vi "goal_loop.vi"(8 "error in":errorcluster, 11 "Micron config":T1) -> (0 "error out":errorcluster)   [LabVIEW 2014]
uses:
  initialization/micron_config.ctl
  manipulator/squiggle/Host/i2c_interface.ctl
  manipulator/squiggle/Host/fpga_reference.ctl
  testing/Micron params.ctl
  testing/stimulus.ctl
  testing/injection_point.ctl
  goal_loop_parms.ctl
  testing/mode_conrols.ctl
  testing/manipulator_cal.ctl
  asap/labview/testing/probe_calibration.ctl
  host/network_params.ctl
  cancellation/sq_control_params.ctl
  cancellation/decoupled_gain.ctl
  cancellation/estimation_controls.ctl
  <vilib>/Platform/TimedLoop/XDataNode/timing_clust.ctl
  <vilib>/Platform/TimedLoop/XDataNode/nitl_modes.ctl
  <vilib>/Platform/TimedLoop/XDataNode/wakeup.ctl
  testing/stimulate.vi
  <vilib>/Analysis/baseanly.llb/A x B.vi
  <vilib>/Analysis/baseanly.llb/A x Vector.vi
  initialization/micron_globals.vi
  <vilib>/Platform/TimedLoop/XDataNode/XDataNode.xnode
  <vilib>/Platform/TimedLoop/XDataNode/XDNodeRunTimeDep.lvlib
panel:
  in  "Sampling frequency":sgl=1000.0
  # "Locals:"
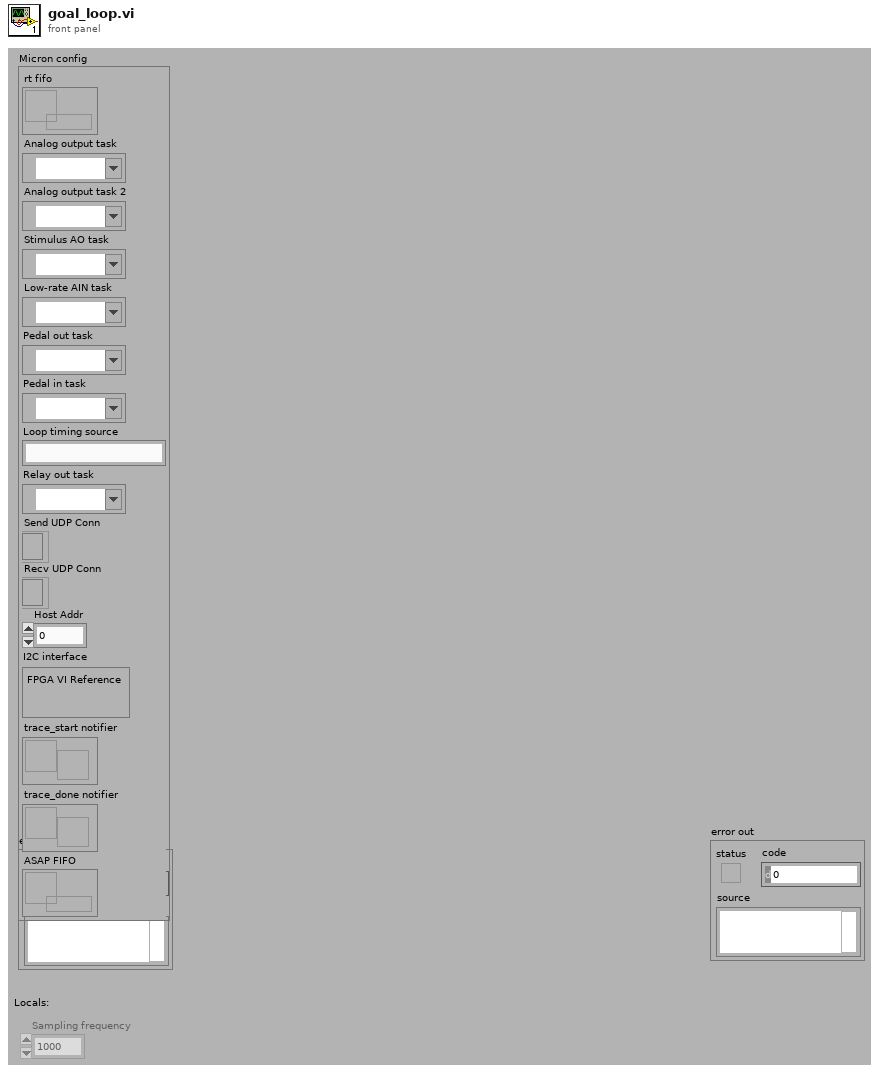
[diagram p1: front panel]
types:
  T1 = typedef "micron_config.ctl" = cluster{"rt fifo":refnum<k33>, "Analog output task":refnum<k21>, "Analog output task 2":refnum<k21>, "Stimulus AO task":refnum<k21>, "Low-rate AIN task":refnum<k21>, "Pedal out task":refnum<k21>, "Pedal in task":refnum<k21>, "Loop timing source":string, "Relay out task":refnum<k21>, "Send UDP Conn":refnum<k16>, "Recv UDP Conn":refnum<k16>, "Host Addr":u32, "I2C interface":T2, "trace_start notifier":refnum<notifier>, "trace_done notifier":refnum<notifier>, "ASAP FIFO":refnum<k33>}
  T2 = typedef "i2c_interface.ctl" = cluster{"FPGA VI Reference":T3}
  T3 = typedef "fpga_reference.ctl" = refnum<k20>
  T4 = typedef "Micron params.ctl" = cluster{"Stimulus":T5, "Goal Filter A":T7, "Mode controls":T8, "Manipulator type":enum16{"Current piezo", "Voltage piezo"}, "Manipulator calibration":T9, "Network":T11, "Goal Filter B":T7, "Cancellation":T12, "Transition time":sgl, "Estimation":T14}
  T5 = typedef "stimulus.ctl" = cluster{"Type":enum16{"Off", "Step", "Sine", "Triangle", "Arbitrary"}, "Phase":dbl, "Amplitude":sgl[], "Injection point":T6, "Closed loop":bool, "Offset":sgl[], "Tip -> world":bool, "Frequency":dbl, "Length":dbl}
  T6 = typedef "injection_point.ctl" = enum16{"Total pose", "V limiter", "Goal ", "Link position", "KF link position", "Inverse kin", "Link goal", "Link error", "Controller", "Output", "Drive", "Light"}
  T7 = typedef "goal_loop_parms.ctl" = cluster{"Speedup max":sgl, "Speedup thresh":sgl, "Speedup nonlin":sgl, "Filters":cluster{"Lower Fc":sgl, "Lower Q":sgl, "Scale factor":sgl, "Upper Fc":sgl, "Upper Q":sgl, "V limit":sgl, "V limit range":sgl}[]}
  T8 = typedef "mode_conrols.ctl" = cluster{"Hold":bool, "Cancellation":bool, "Goal filter":bool, "Trigger":bool}
  T9 = typedef "manipulator_cal.ctl" = cluster{"Tool offsets":sgl[][], "Tip light calibration":T10, "Handle light calibration":T10, "Base pivots":sgl[][], "Output pivots":sgl[][], "Length center":sgl, "Workspace height":sgl[], "Workspace diameter":sgl[], "Linearization":sgl[][], "Stack travel":sgl, "Saturation pos":sgl, "Inverse filters":cluster{"filter structure":enum32{"IIR 2nd Order", "IIR 4th Order"}, "Reverse Coefficients":dbl[], "Forward Coefficients":dbl[]}[]}
  T10 = typedef "probe_calibration.ctl" = sgl[][]
  T11 = typedef "network_params.ctl" = cluster{"Remote Host":string, "Send Status":bool, "Send Port":u16, "Recv Commands":bool, "Recv Port":u16}
  T12 = typedef "sq_control_params.ctl" = cluster{"KP":T13, "KI":sgl, "KD":T13, "Max vel":sgl, "Max acc":sgl, "Int error limit":sgl, "RCM gain":sgl, "Bypass":bool, "Degraded gain":sgl}
  T13 = typedef "decoupled_gain.ctl" = cluster{"XY":sgl, "Rxy":sgl, "Z":sgl, "Rz":sgl}
  T14 = typedef "estimation_controls.ctl" = cluster{"Link":cluster{"Measure noise":dbl[], "Process noise":dbl[], "Alt process noise":dbl[], "Alt turnoff cycles":i32, "Innovation limit":dbl[], "Residue threshold":dbl, "Enable":bool}, "Handle":cluster{"Measure noise":dbl[], "Process noise":dbl[], "State limits":dbl[], "Innovation limit":dbl[], "Prediction Lookahead":sgl, "Enable":bool}}
  T15 = typedef "XDNodeRunTimeDep.lvlib/timing_clust.ctl" = cluster{"Expected End [f-1]":u64, "Actual End [f-1]":u64, "Finished Late? [f-1]":bool, "Expected End [i-1]":u64, "Actual End [i-1]":u64, "Finished Late? [i-1]":bool, "Expected Start [i]":u64, "Actual Start [i]":u64, "Expected Start [f]":u64, "Actual Start [f]":u64, "Source Name":string, "Structure Name":string, "Period":i64, "Deadline":i64, "Offset":i64, "Start":i64, "Priority":i32, "Timeout":i32, "Mode":T16, "Wakeup Reason":T17, "Error":errorcluster, "Source Type":string, "Secondary Source Type":string, "Global End Time":u64, "Global Start Time":u64, "Frame Duration":u64, "Iteration Duration":u64, "Assigned CPU":i32, "I/O Scan Engine Mode":u32}
  T16 = typedef "XDNodeRunTimeDep.lvlib/nitl_modes.ctl" = enum32{"No Change", "Process missed periods, maintain original phase", "Discard missed periods, maintain original phase", "Process missed periods, ignore original phase", "Discard missed periods, ignore original phase"}
  T17 = typedef "XDNodeRunTimeDep.lvlib/wakeup.ctl" = enum32{"Normal", "Aborted", "Asynchronous wakeup", "Timing source error", "Timed loop error", "Timeout"}
  T18 = cluster{"Lower Fc":sgl, "Lower Q":sgl, "Scale factor":sgl, "Upper Fc":sgl, "Upper Q":sgl, "V limit":sgl, "V limit range":sgl}[]
  T19 = typedef "NI_Matrix.lvlib/RealMatrix.ctl" = dbl[][]
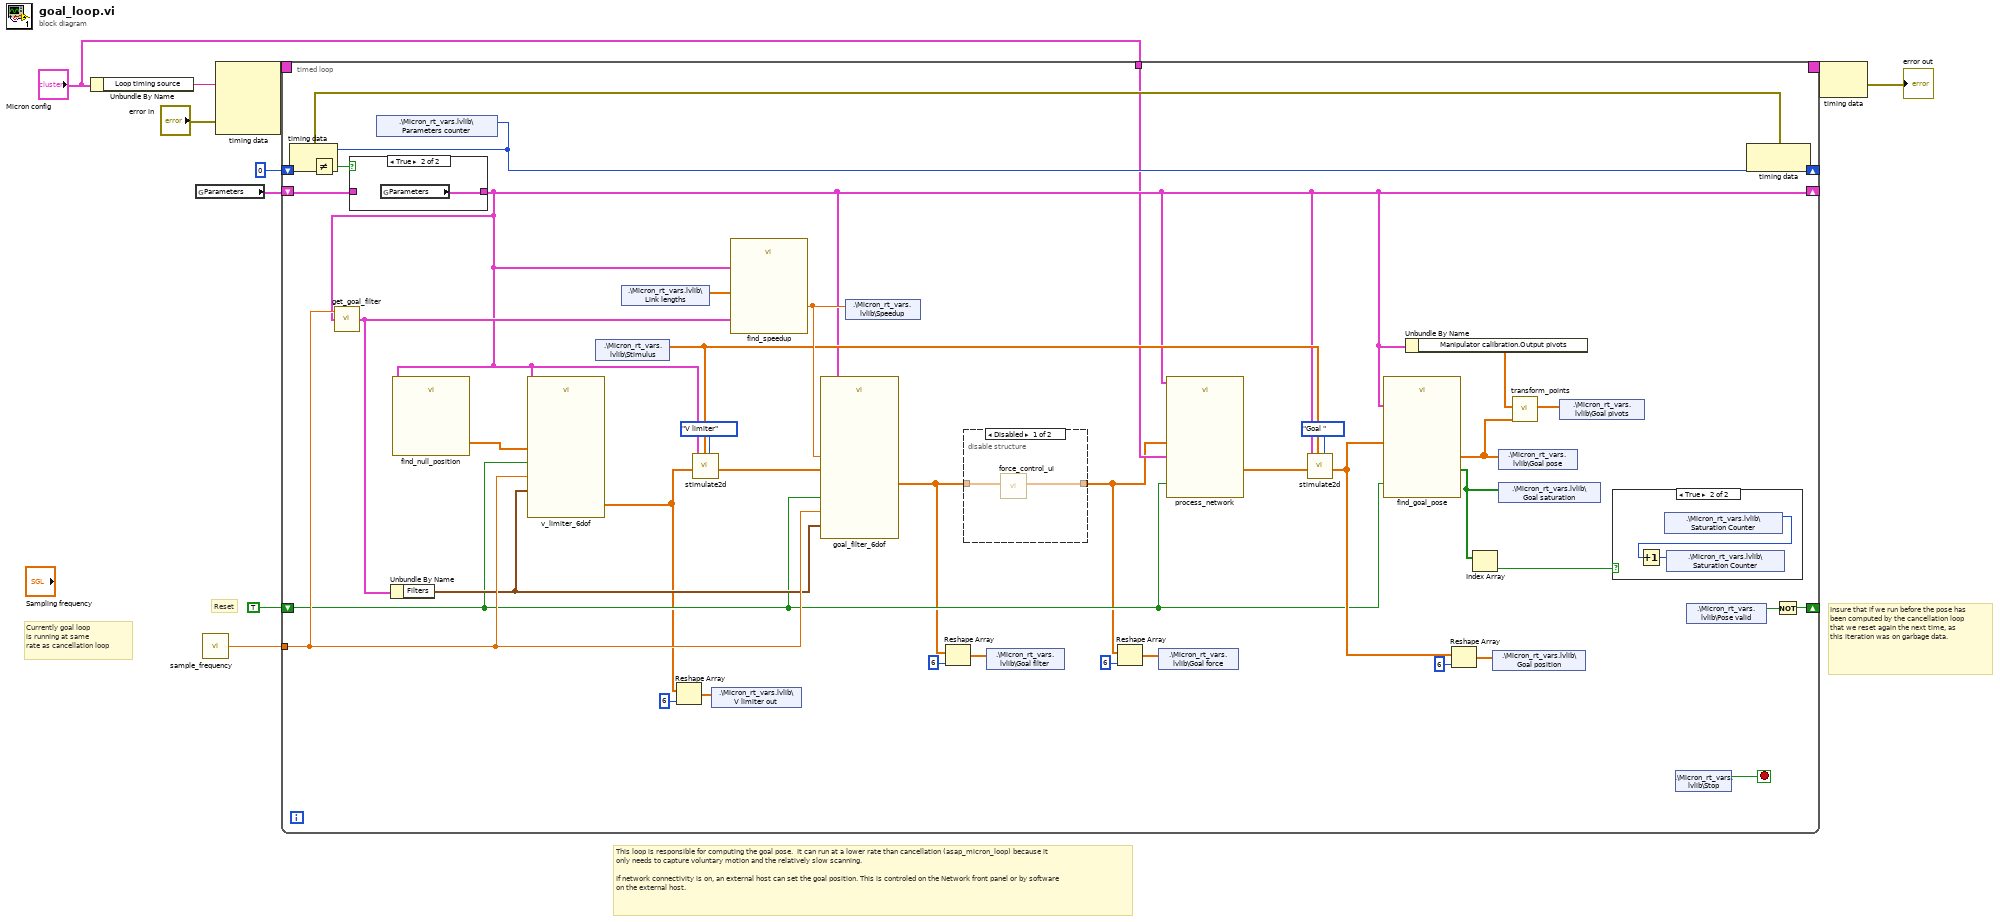
[diagram p0: block diagram]
diagram:
  # "Currently goal loop\nis running at same\nrate as cancellation loop"
  # "Reset"
  # "Insure that if we run before the pose has been computed by the cancellation loop that we reset again the next time, as this iteration was on garbage data."
  # "This loop is responsible for computing the goal pose.  It can run at a lower rate than cancellation (asap_micron_loop) because it only needs to capture voluntary motion and the relatively slow scanning.\n\nIf network connectivity is on, an external host can set the goal position. This is controled on the Network front panel or by software on the external host."
  n1 = Unbundle By Name("Micron config") -> ("Loop timing source"=w2:string)
  n2 = global read "micron_globals.vi" "Parameters"() -> (w4:T4)
  n3 = call "sample_frequency.vi"() -> ("Sample frequency"=w3:dbl)
  n4 = node-c288(w2, "error in") -> (w10:T15)  [unwired: 2 out]
  n5 = timed-loop {
    timing: w10 -> [_]
    timing-out: [_] -> w9
    shift-right: [w46] -> _
    shift-left: TRUE ("Saturation") -> [w19]
    shift-right: [w23] -> _
    shift-left: w4 -> [w42]
    shift-right: [w43] -> _
    shift-left: u32 0 ("Parameters counter") -> [w44]
    tunnel: w3 -> [w38]
    tunnel: "Micron config" -> [w20]
    stop <- w48 stop-if-true
    n6 = node-c288() -> (w49:errorcluster)  [unwired: 1 out]
    n7 = shared-variable ".\\Micron_rt_vars.lvlib\\Parameters counter"() -> (w43:u32)  [unwired: 2 out]
    n8 = Not Equal?(x=w43, y=w44) -> (x != y?=w45:bool)
    n9 = case shown="True" w45 {
      tunnel: [w55 w56] -> w23
      tunnel: w42 -> [w55 _]
      frame False {
      }
      frame True {
        n10 = global read "micron_globals.vi" "Parameters"() -> (w56:T4)
      }
    }
    n11 = call "get_goal_filter.vi"("Parameters"=w23, "Sampling frequency"=w38) -> ("Goal loop params"=w35:T7)  [unwired: 3 out]
    n12 = Unbundle By Name(w35) -> ("Filters"=w32:T18)
    n13 = call "find_null_position.vi"("Parameters"=w23) -> ("Null position"=w18:sgl[][])  [unwired: 1 in, 9 out]
    n14 = call "v_limiter_6dof.vi"("Filters"=w32, "Sampling frequency"=w38, "Reset"=w19, "Input"=w18, "Parameters"=w23) -> ("Goal position out"=w17:sgl[][])  [unwired: 1 in]
    n15 = shared-variable ".\\Micron_rt_vars.lvlib\\Stimulus"() -> (w28:sgl[])  [unwired: 2 out]
    n16 = shared-variable ".\\Micron_rt_vars.lvlib\\Link lengths"() -> (w41:sgl[])  [unwired: 2 out]
    n17 = Reshape Array(w17, 6 ("dimension size")) -> (w33:sgl[])
    n18 = call "stimulate2d.vi"("Injection point"=injection_point."V limiter", "Stimulus"=w28, "Input"=w17, "Parameters"=w23) -> ("Output"=w36:sgl[][])  [unwired: 6 in]
    n19 = shared-variable ".\\Micron_rt_vars.lvlib\\V limiter out"(w33) -> ()  [unwired: 2 out]
    n20 = call "find_speedup.vi"("Parameters"=w23, "Goal Filter"=w35, "Stack positions"=w41) -> ("Speedup"=w40:sgl)  [unwired: 8 out]
    n21 = call "goal_filter_6dof.vi"("Filters"=w32, "Speedup"=w40, "Sampling frequency"=w38, "Reset"=w19, "Input"=w36, "Parameters"=w23) -> ("Goal position out"=w14:sgl[][])
    n22 = shared-variable ".\\Micron_rt_vars.lvlib\\Speedup"(w40) -> ()  [unwired: 2 out]
    n23 = Reshape Array(w14, 6 ("dimension size")) -> (w16:sgl[])
    n24 = disable-structure shown="Disabled" {
      disable-tunnel: w14 -> [w51 w52]
      disable-tunnel: [w50 w52] -> w11
      frame Disabled {
        n25 = call "force_control_ui.vi"("Goal Position IN"=w51) -> ("Goal Position OUT"=w50:sgl[][])  [unwired: 9 in]
      }
      frame Enabled {
      }
    }
    n26 = shared-variable ".\\Micron_rt_vars.lvlib\\Goal filter"(w16) -> ()  [unwired: 2 out]
    n27 = Reshape Array(w11, 6 ("dimension size")) -> (w12:sgl[])
    n28 = shared-variable ".\\Micron_rt_vars.lvlib\\Goal force"(w12) -> ()  [unwired: 2 out]
    n29 = call "process_network.vi"("Micron config"=w20, "Reset"=w19, "Goal position in"=w11, "Parameters"=w23) -> ("Goal position out"=w31:sgl[][])  [unwired: 7 in]
    n30 = call "stimulate2d.vi"("Injection point"=injection_point."Goal ", "Stimulus"=w28, "Input"=w31, "Parameters"=w23) -> ("Output"=w27:sgl[][])  [unwired: 6 in]
    n31 = call "find_goal_pose.vi"("Reset"=w19, "Parameters"=w23, "Goal position"=w27) -> ("Saturation"=w22:bool[], "Goal pose"=w24:T19)  [unwired: 7 in]
    n32 = Unbundle By Name(w23) -> ("Manipulator calibration.Output pivots"=w26:sgl[][])
    n33 = Reshape Array(w27, 6 ("dimension size")) -> (w29:sgl[])
    n34 = Index Array(array=w22) -> (element=w21:bool)  [unwired: 1 in]
    n35 = shared-variable ".\\Micron_rt_vars.lvlib\\Goal position"(w29) -> ()  [unwired: 2 out]
    n36 = shared-variable ".\\Micron_rt_vars.lvlib\\Goal pose"(w24) -> ()  [unwired: 1 in, 1 out]
    n37 = shared-variable ".\\Micron_rt_vars.lvlib\\Goal saturation"(w22) -> ()  [unwired: 1 in, 1 out]
    n38 = call "transform_points.vi"("Transform"=w24, "Points"=w26) -> ("Transformed points"=w25:sgl[][])  [unwired: 9 in]
    n39 = shared-variable ".\\Micron_rt_vars.lvlib\\Goal pivots"(w25) -> ()  [unwired: 2 out]
    n40 = case shown="True" w21 {
      frame False {
      }
      frame True {
        n41 = shared-variable ".\\Micron_rt_vars.lvlib\\Saturation Counter"() -> (w53:u32)  [unwired: 2 out]
        n42 = Increment(x=w53) -> (x+1=w54:u32)
        n43 = shared-variable ".\\Micron_rt_vars.lvlib\\Saturation Counter"(w54) -> ()  [unwired: 2 out]
      }
    }
    n44 = shared-variable ".\\Micron_rt_vars.lvlib\\Stop"() -> (w48:bool)  [unwired: 2 out]
    n45 = shared-variable ".\\Micron_rt_vars.lvlib\\Pose valid"() -> (w47:bool)  [unwired: 2 out]
    n46 = node-c288(w49) -> ()  [unwired: 1 out]
    n47 = Not(x=w47) -> (.not. x?=w46:bool)
  }
  n48 = node-c288(w9) -> (→"error out":errorcluster)
